vi "write.vi"(5 "remote transmission request? (F)":bool, 7 "extended id? (F)":bool, 8 "error in (no error)":errorcluster, 9 "data":u8[](array[numeric]) format="%x", 10 "id":u32 format="%x", 11 "channel":u16 format="%x") -> (0 "error out":errorcluster)   [LabVIEW 2024, in "atsj peakcan basic.lvlib"]
doc: "Writes a CAN message through a PeakCAN <b>channel</b>."
uses:
  atsj peakcan basic.lvlib
  support/x64/PCANBasic.dll
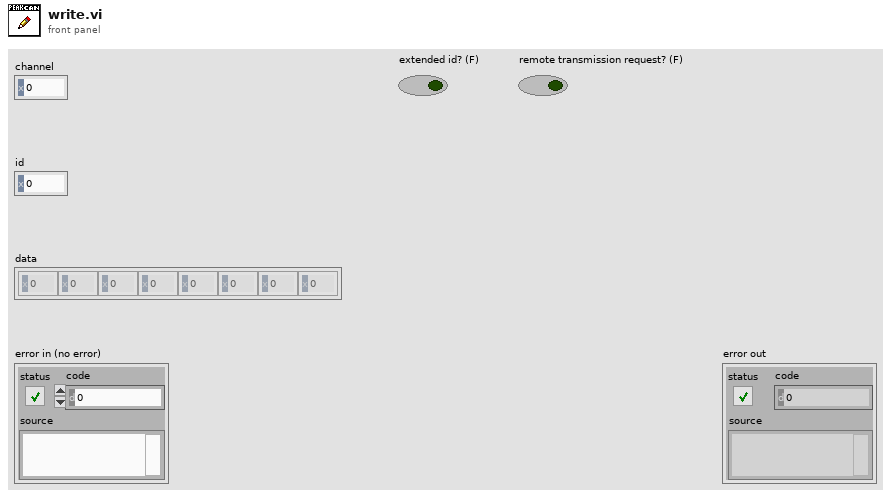
[diagram p1: front panel]
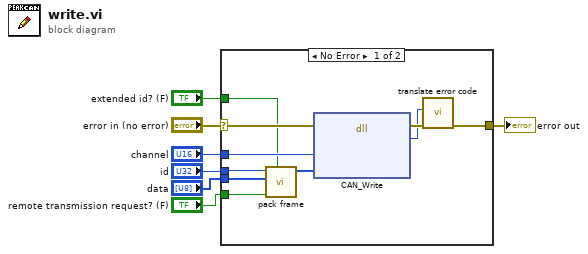
[diagram p0: block diagram]
diagram:
  n1 = case shown="No Error" "error in (no error)" {
    selector: "error in (no error)" -> [w13 w18]
    tunnel: "id" -> [w11 _]
    tunnel: "channel" -> [w17 _]
    tunnel: [w14 w18] -> w5
    tunnel: "data" -> [w10 _]
    tunnel: "remote transmission request? (F)" -> [w9 _]
    tunnel: "extended id? (F)" -> [w8 _]
    frame No Error {
      n2 = call "pack frame.vi"("extended id?"=w8, "remote transmission request? (F)"=w9, "data"=w10, "id"=w11) -> ("frame"=w12:u8[])  [unwired: 7 in]
      n3 = dll-call lib="C:/atsj/plateau/atsj-peakcan-basic-for-labview/src/support/x64/PCANBasic.dll" fn="CAN_Write" ("write")(error in=w13, "Channel"=w17, "MessageBuffer"=w12) -> (error out=w16:errorcluster, "Status"=w15:u32)  [unwired: 4 in, 1 out]
      n4 = call "translate error code.vi"("error in (no error)"=w16, "error code"=w15) -> ("error out"=w14:errorcluster)  [unwired: 9 in]
    }
    frame Error {
    }
  }
  "error out" <- w5
